vi "IDS Preview Capture.vi"(6 "Pixel Size (µm)":dbl=-1.0, 8 "Image Ref":T1, 9 "IDS Camera Ref":refnum<k24>, 10 "IDS Actions":T2, 11 "IDS Notifier":refnum<notifier>) -> (0 "Error":errorcluster, 3 "IDS Notifier":refnum<notifier>)   [LabVIEW 2025]
uses:
  IDS Controls/IDS Actions.ctl
  IDS Controls/IDS Notifier Element.ctl
  IDS Controls/IDS Parameters.ctl
  IDS Controls/IDS Parameter List.ctl
  IDS Controls/IDS ROI.ctl
  <vilib>/vision/Image Controls.llb/IMAQ Image.ctl
  C:/Users/Photonics03/Documents/Microscope-Control/Device Library/Cameras/IDS/IDS LabView Examples/LabVIEW/ueye.NET/uEyeDotNet.dll
  IDS LabView Examples/LabVIEW/ueye.NET/uEyeDotNet.dll
  Tools/TIFF Image Read and Write/ImageJ TIF Type Defs/TIF Write Image Information.ctl
  Camera Controls/Camera IMAQ Key Info.ctl
  <vilib>/vision/NI_Vision_Development_Module.lvlib
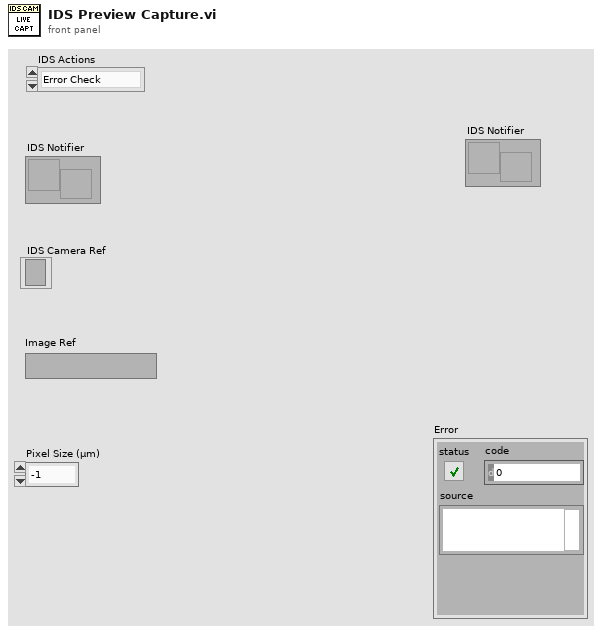
[diagram p1: front panel]
types:
  T1 = typedef "IMAQ Image.ctl" = refnum<image>
  T2 = typedef "IDS Actions.ctl" = enum16{"Error Check", "Initialize", "Preview", "Record", "Abort", "Record Settings", "Set Parameter", "Get Parameter", "Set ROI", "Get ROI", "Status", "Quit"}
  T3 = typedef "Image Type" = u32
  T4 = typedef "Camera IMAQ Key Info.ctl" = cluster{"Frame":u32, "Sensor Height":i32, "Sensor Width":i32, "ROI Height":i32, "ROI Width":i32, "ROI Enable?":bool, "Bit per Pixel":u8}
  T5 = typedef "TIF Write Image Information.ctl" = cluster{"Image Width (Pixels)":u32, "Image Height (Pixels)":u32, "Pixel Width (µm)":dbl, "Pixel Height (µm)":dbl, "Bits Per Sample (e.g. 16)":u32, "No. of Frames":u32, "No. of Slices":u32, "Time Step (sec)":dbl, "Z Step (µm)":dbl}
  T6 = typedef "IDS Notifier Element.ctl" = cluster{"IDS Actions":T2, "Received?":bool, "IDS Parameter":T7, "IDS ROI":T9, "Running?":bool, "File Path":path, "# of frames":u32, "Image Ref":T1, "Error":errorcluster, "Binning":i32}
  T7 = typedef "IDS Parameters.ctl" = cluster{"Parameter":T8, "Value":dbl}
  T8 = typedef "IDS Parameter List.ctl" = enum16{"Exposure Time (s)", "Binning"}
  T9 = typedef "IDS ROI.ctl" = cluster{"H Offset":i32, "V Offset":i32, "H Width":i32, "V Width":i32}
  T10 = enum16{"big-endian, network order", "native, host order", "little-endian"}
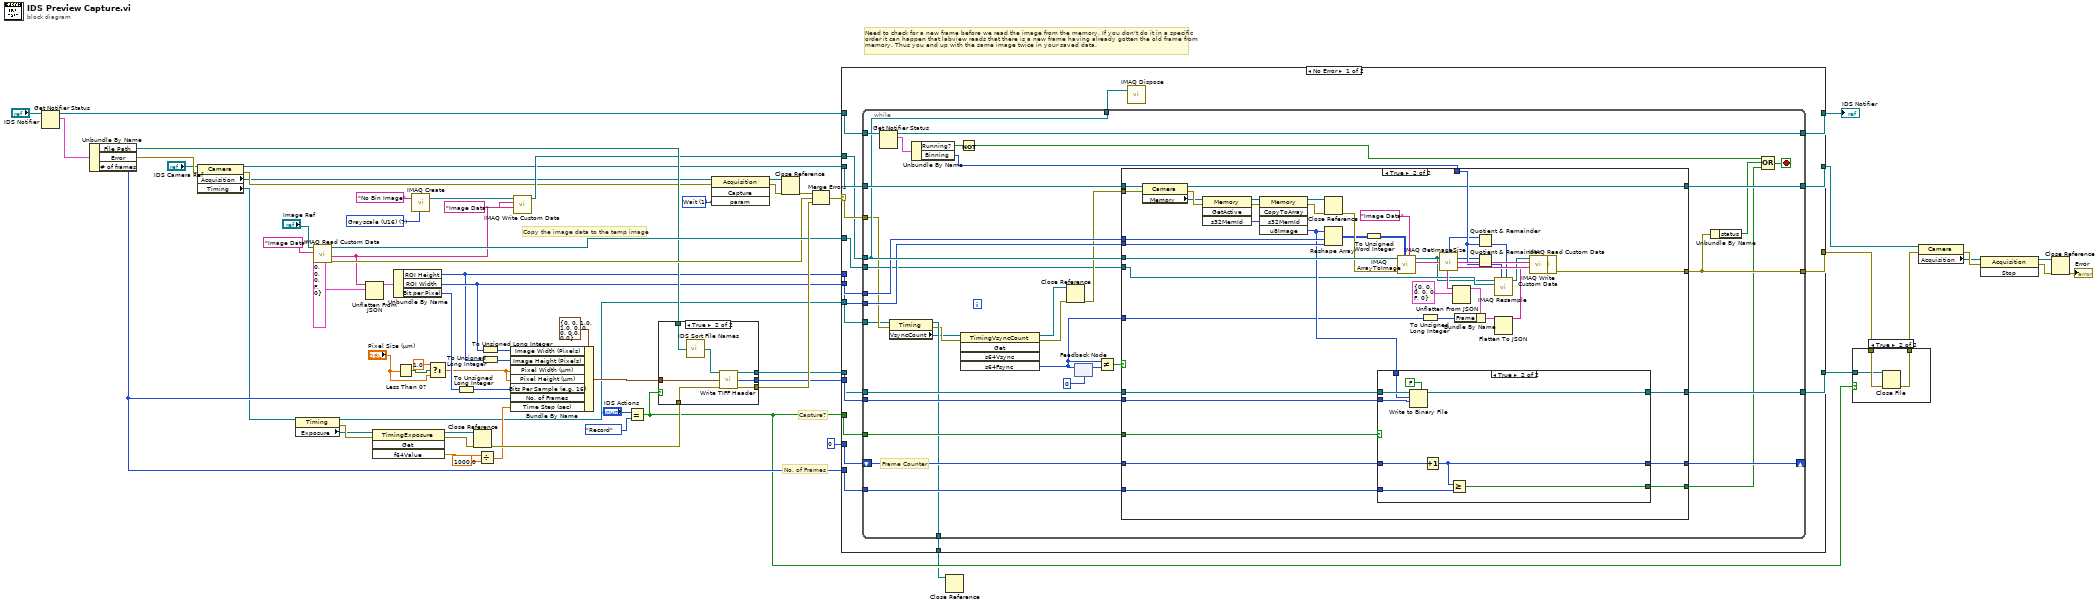
[diagram p0: block diagram]
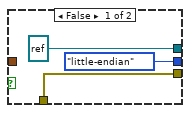
[diagram p3: hidden frame]
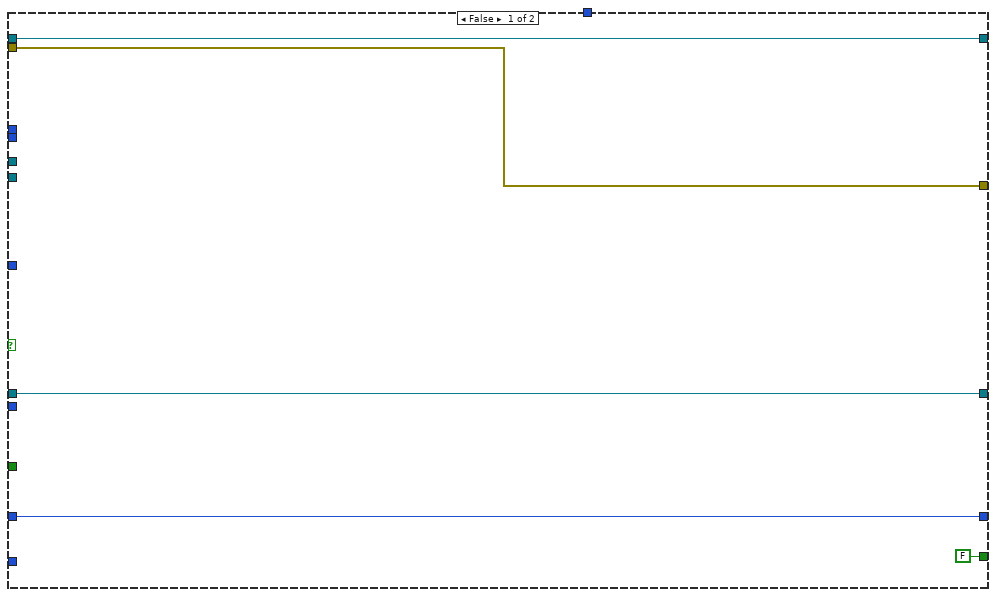
[diagram p4: hidden frame]
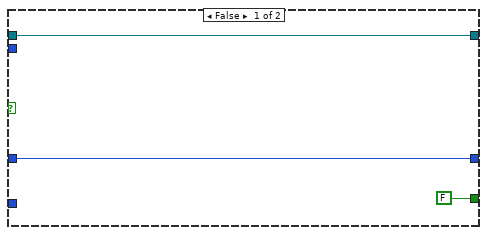
[diagram p5: hidden frame]
diagram:
  w15 = T3 7 items=["Grayscale (U8)", "Grayscale (I16)", "Grayscale (SGL)", "Complex (CSG)", "RGB (U32)", "HSL (U32)", "RGB (U64)", "Grayscale (U16)"] ("Image Type")
  w29 = 1 items=["DontWait"=0, "Wait"=1, "Force"=16384] ("param")
  # "Copy the image data to the temp image"
  # "Need to check for a new frame before we read the image from the memory. If you don't do it in a specific\norder it can happen that labview reads that there is a new frame having already gotten the old frame from\nmemory. Thus you end up with the same image twice in your saved data."
  # "Capture?"
  # "No. of Frames"
  n1 = Get Notifier Status(notifier="IDS Notifier") -> (notifier out=w56:refnum<notifier>, current notification=w55:T6)  [unwired: 1 in, 3 out]
  n2 = Unbundle By Name(w55) -> ("File Path"=w36:path, "Error"=w6:errorcluster, "# of frames"=w37:u32)
  n3 = property class="Camera"(reference="IDS Camera Ref", error in=w6) -> (reference out=w10:refnum<k24>, error out=w9:errorcluster, "Acquisition"=w8:refnum<k24>, "Timing"=w7:refnum<k24>)
  n4 = property class="Timing"(reference=w7) -> (reference out=w13:refnum<k24>, error out=w12:errorcluster, "Exposure"=w11:refnum<k24>)  [unwired: 1 in]
  n5 = call "IMAQ Read Custom Data"("Key"="Image Data", "Image"="Image Ref") -> ("error out"=w43:errorcluster, "Custom Data Out"=w41:string, "Image (duplicate)"=w44:T1)  [unwired: 7 in]
  n6 = Unflatten From JSON(JSON string=w41, type and defaults=T4 {"Frame"=0, "Sensor Height"=0, "Sensor Width"=0, "ROI Height"=0, "ROI Width"=0, "ROI Enable?"=FALSE, "Bit per Pixel"=0} ("Camera IMAQ Key Info")) -> (value=w40:T4)  [unwired: 5 in, 1 out]
  n7 = invoke class="TimingExposure" method="Get"(reference=w11, error in=w12) -> (reference out=w47:refnum<k24>, error out=w46:errorcluster, "f64Value"=w26:dbl)  [unwired: 2 in, 1 out]
  n8 = Unbundle By Name(w40) -> ("ROI Height"=w34:i32, "ROI Width"=w35:i32, "Bit per Pixel"=w28:u8)
  n9 = Less Than 0?(x="Pixel Size (µm)") -> (x < 0?=w21:bool)
  n10 = call "IMAQ Create"("Image Name"="No Bin Image", "Image Type"=w15) -> ("New Image"=w17:T1)  [unwired: 3 in, 1 out]
  n11 = Select(t=1.0, s=w21, f="Pixel Size (µm)") -> (s? t:f=w22:dbl)
  n12 = To Unsigned Long Integer(number=w28) -> (unsigned 32bit integer=w23:u32)
  n13 = Close Reference(reference=w47, error in (no error)=w46) -> (error out=w45:errorcluster)
  n14 = Divide(x=w26, y=1000.0) -> (x/y=w24:dbl)
  n15 = To Unsigned Long Integer(number=w35) -> (unsigned 32bit integer=w50:u32)
  n16 = To Unsigned Long Integer(number=w34) -> (unsigned 32bit integer=w49:u32)
  n17 = Bundle By Name(cluster=T5 {"Image Width (Pixels)"=0, "Image Height (Pixels)"=0, "Pixel Width (µm)"=1.0, "Pixel Height (µm)"=1.0, "Bits Per Sample (e.g. 16)"=0, "No. of Frames"=0, "No. of Slices"=0, "Time Step (sec)"=0.0, "Z Step (µm)"=0.0} ("Image Info"), "Image Width (Pixels)"=w50, "Image Height (Pixels)"=w49, "Pixel Width (µm)"=w22, "Pixel Height (µm)"=w22, "Bits Per Sample (e.g. 16)"=w23, "No. of Frames"=w37, "Time Step (sec)"=w24) -> (w51:T5)
  n18 = call "IMAQ Write Custom Data"("Custom Data In"=w41, "Key"="Image Data", "Image"=w17) -> ("Image Out"=w18:T1)  [unwired: 7 in, 1 out]
  n19 = Equal?(x="IDS Actions", y=IDS_Actions."Record") -> (x = y?=w31:bool)
  n20 = case shown="True" w31 {
    tunnel: w51 -> [_ w77]
    tunnel: w36 -> [_ w72]
    tunnel: [w70 w76] -> w48
    tunnel: w45 -> [w70 w75]
    tunnel: [refnum<file> refnum ("File Ref") w74] -> w38
    tunnel: [T10."little-endian" ("Byte Order") w73] -> w39
    frame False {
    }
    frame True {
      n21 = call "IDS Sort File Names.vi"("Requested File Path"=w72) -> ("Resulting File Path"=w71:path)  [unwired: 14 in]
      n22 = call "Write TIFF Header.vi"("File Path"=w71, "Image Info"=w77, "Error"=w75) -> ("File Ref"=w74:refnum<file>, "Byte Order"=w73:T10, "Error"=w76:errorcluster)  [unwired: 10 in]
    }
  }
  n23 = invoke class="Acquisition" method="Capture"(reference=w8, error in=w9, "param"=w29) -> (reference out=w67:refnum<k24>, error out=w66:errorcluster)  [unwired: 1 in, 2 out]
  n24 = Close Reference(reference=w67, error in (no error)=w66) -> (error out=w65:errorcluster)
  n25 = Merge Errors(w65, w43, w48) -> (w64:errorcluster)
  n26 = case shown="No Error" w64 {
    selector: w64 -> [w92 w197]
    tunnel: w56 -> [w96 w195]
    tunnel: [w91 w195] -> w59
    tunnel: w10 -> [w95 w196]
    tunnel: w34 -> [w94 _]
    tunnel: w35 -> [w93 _]
    tunnel: w44 -> [w80 _]
    tunnel: [w90 w197] -> w32
    tunnel: [w89 w196] -> w1
    tunnel: w31 -> [w88 _]
    tunnel: w39 -> [w87 _]
    tunnel: w38 -> [w86 w194]
    tunnel: w37 -> [w85 _]
    tunnel: [w84 w194] -> w33
    tunnel: w13 -> [w83 w193]
    tunnel: [w82 w193] -> w30
    tunnel: u32 0 ("s64Fsync") -> [w81 _]
    tunnel: w18 -> [w79 _]
    frame No Error {
      n27 = while {
        tunnel: w96 -> [w131]
        tunnel: w95 -> [w130]
        tunnel: w94 -> [w127]
        tunnel: w93 -> [w126]
        tunnel: w92 -> [w98]
        tunnel: [w129] -> w89
        tunnel: w79 -> [w128]
        tunnel: [w125] -> w91
        tunnel: [w124] -> w90
        tunnel: w88 -> [w110]
        tunnel: w87 -> [w121]
        tunnel: w86 -> [w122]
        tunnel: w85 -> [w123]
        tunnel: [w117] -> w84
        tunnel: w83 -> [w97]
        tunnel: [w101] -> w82
        shift-right: [w112] -> _
        shift-left: w81 -> [w113]
        tunnel: w80 -> [w105]
        tunnel: [w128] -> w78
        stop <- w118 stop-if-true
        # "Frame Counter"
        n28 = Get Notifier Status(notifier=w131) -> (notifier out=w125:refnum<notifier>, current notification=w102:T6)  [unwired: 1 in, 3 out]
        n29 = property class="Timing"(reference=w97, error in=w98) -> (reference out=w101:refnum<k24>, error out=w100:errorcluster, "VsyncCount"=w99:refnum<k24>)
        n30 = Unbundle By Name(w102) -> ("Running?"=w104:bool, "Binning"=w103:i32)
        n31 = Not(x=w104) -> (.not. x?=w120:bool)
        n32 = invoke class="TimingVsyncCount" method="Get"(reference=w99, error in=w100) -> (reference out=w106:refnum<k24>, error out=w108:errorcluster, "s64Fsync"=w114:i64)  [unwired: 3 in, 2 out]
        n33 = Close Reference(reference=w106, error in (no error)=w108) -> (error out=w107:errorcluster)
        n34 = feedback #1(i64 0 ("s64Fsync")) -> (w115:i64)
        n35 = feedback-in #1(w114) -> ()
        n36 = Not Equal?(x=w114, y=w115) -> (x != y?=w109:bool)
        n37 = case shown="True" w109 {
          tunnel: w130 -> [w136 w137]
          tunnel: [w136 w141] -> w129
          tunnel: w128 -> [_ w175]
          tunnel: w127 -> [_ w174]
          tunnel: w126 -> [_ w173]
          tunnel: [w135 w171] -> w124
          tunnel: w123 -> [_ w162]
          tunnel: w122 -> [w132 w161]
          tunnel: w121 -> [_ w160]
          tunnel: [w132 w156] -> w117
          tunnel: w114 -> [_ w154]
          tunnel: w107 -> [w135 w138]
          tunnel: w113 -> [w134 w153]
          tunnel: [w134 w152] -> w112
          tunnel: [FALSE w151] -> w111
          tunnel: w110 -> [_ w150]
          tunnel: w105 -> [_ w149]
          tunnel: w103 -> [_ w146]
          frame False {
          }
          frame True {
            w168 = "Image Data" ("Key")
            n38 = property class="Camera"(reference=w137, error in=w138) -> (reference out=w141:refnum<k24>, error out=w140:errorcluster, "Memory"=w139:refnum<k24>)
            n39 = invoke class="Memory" method="GetActive"(reference=w139, error in=w140) -> (reference out=w180:refnum<k24>, error out=w178:errorcluster, "s32MemId"=w179:i32)  [unwired: 2 in, 1 out]
            n40 = invoke class="Memory" method="CopyToArray"(reference=w180, error in=w178, "s32MemId"=w179) -> (reference out=w177:refnum<k24>, error out=w176:errorcluster, "u8Image"=w157:u8[])  [unwired: 2 in, 2 out]
            n41 = Close Reference(reference=w177, error in (no error)=w176) -> (error out=w172:errorcluster)
            n42 = Reshape Array(w157, w174, w173) -> (w158:u8[][])
            n43 = To Unsigned Word Integer(number=w158) -> (unsigned 16bit integer=w159:u16[][])
            n44 = case shown="True" w150 {
              tunnel: w162 -> [_ w192]
              tunnel: w161 -> [w183 w188]
              tunnel: w160 -> [_ w191]
              tunnel: [w183 w189] -> w156
              tunnel: w157 -> [_ w187]
              tunnel: w153 -> [w182 w186]
              tunnel: [w182 w185] -> w152
              tunnel: [FALSE w184] -> w151
              frame False {
              }
              frame True {
                n45 = Write to Binary File(file (use dialog)=w188, data=w187, 5:FALSE ("prepend array or string size? (T)"), 9:w191) -> (refnum out=w189:refnum<file>)  [unwired: 2 in, 2 out]
                n46 = Increment(x=w186) -> (x+1=w185:u32)
                n47 = Greater Or Equal?(x=w185, y=w192) -> (x >= y?=w184:bool)
              }
            }
            n48 = call "IMAQ ArrayToImage"("Image Pixels (U16)"=w159, "error in (no error)"=w172, "Image"=w175) -> ("Image Out"=w142:T1)  [unwired: 7 in, 1 out]
            n49 = To Unsigned Long Integer(number=w154) -> (unsigned 32bit integer=w155:u32)
            n50 = call "IMAQ GetImageSize"("Image"=w142) -> ("Y Resolution"=w144:i32, "X Resolution"=w143:i32)  [unwired: 3 in, 1 out]
            n51 = Quotient & Remainder(x=w143, y=w146) -> (floor(x/y)=w147:i32)  [unwired: 1 out]
            n52 = Quotient & Remainder(x=w144, y=w146) -> (floor(x/y)=w145:i32)  [unwired: 1 out]
            n53 = call "IMAQ Resample"("X Resolution"=w147, "Y Resolution"=w145, "Image Dst"=w149, "Image Src"=w142) -> ("Image Dst Out"=w148:T1)  [unwired: 6 in, 1 out]
            n54 = call "IMAQ Read Custom Data"("Key"=w168, "Image"=w148) -> ("error out"=w169:errorcluster, "Custom Data Out"=w167:string, "Image (duplicate)"=w170:T1)  [unwired: 7 in]
            n55 = Unflatten From JSON(JSON string=w167, type and defaults=T4 {"Frame"=0, "Sensor Height"=0, "Sensor Width"=0, "ROI Height"=0, "ROI Width"=0, "ROI Enable?"=FALSE, "Bit per Pixel"=0} ("Camera IMAQ Key Info")) -> (value=w165:T4)  [unwired: 5 in, 1 out]
            n56 = Bundle By Name(cluster=w165, "Frame"=w155) -> (w164:T4)
            n57 = Flatten To JSON(anything=w164) -> (JSON string=w163:string)  [unwired: 2 in, 1 out]
            n58 = call "IMAQ Write Custom Data"("error in (no error)"=w169, "Custom Data In"=w163, "Key"=w168, "Image"=w170) -> ("error out"=w171:errorcluster)  [unwired: 6 in, 1 out]
          }
        }
        n59 = Unbundle By Name(w124) -> ("status"=w119:bool)
        n60 = Compound Arithmetic op=OR(w120, w119, w111) -> (w118:bool)
      }
      n61 = call "IMAQ Dispose"("Image"=w78) -> ()  [unwired: 5 in, 1 out]
    }
    frame Error {
    }
  }
  "IDS Notifier" <- w59
  n62 = Close Reference(reference=w30) -> ()  [unwired: 1 in, 1 out]
  n63 = case shown="True" w31 {
    tunnel: w33 -> [_ w199]
    tunnel: w32 -> [w198 w201]
    tunnel: [w198 w200] -> w2
    frame False {
    }
    frame True {
      n64 = Close File(refnum=w199, error in=w201) -> (error out=w200:errorcluster)  [unwired: 1 out]
    }
  }
  n65 = property class="Camera"(reference=w1, error in=w2) -> (error out=w4:errorcluster, "Acquisition"=w3:refnum<k24>)  [unwired: 1 out]
  n66 = invoke class="Acquisition" method="Stop"(reference=w3, error in=w4) -> (reference out=w62:refnum<k24>, error out=w61:errorcluster)  [unwired: 1 in, 1 out]
  n67 = Close Reference(reference=w62, error in (no error)=w61) -> (error out=→"Error":errorcluster)
